vi "Write to DB.vi"(8 "error in (no error)":errorcluster, 11 "Database Entry in":refnum<class "Database Entry.lvclass">) -> (0 "error out":errorcluster, 2 "Stack names":string[](array[string]), 3 "Database Entry out":refnum<class "Database Entry.lvclass">)   [LabVIEW 2021, in "Database Entry.lvclass"]
uses:
  Database Entry.lvclass
  Database Entry.lvclass/Database Entry.ctl
  <vilib>/Utility/file.llb/Read Delimited Spreadsheet (string).vi
  <vilib>/Utility/file.llb/Write Delimited Spreadsheet (string).vi
  Components/Stack/Stack.lvclass
panel:
  out "Final name":string
  out "Data cluster":T1={"module or proto"="proto", " geometry"="full", "resolution"="LD", "baselayer"="BA_123", "toplayer"="SI_789", "bl_pos"="1", "tl_pos"="1", "put_pos"="1", "region"="1", "asstray"="1", "comptray"="1", "put"="1", "date"="2024-04-02", "timestart"="1:12:12.442", "timeend"="1:23:45.244", "operator"="cmuperson", "tape"="some", "glue"="some", "stack name"="some", "Adhesive type"="", "Comments"="", "Temperature"="", "Relative Humidity"=""}
  out "error out py":errorcluster
  out "String Out":string="Upload Success"
  in  "error in (no error) py":errorcluster
  # "Debug instructions\n#### The order of values in db_data_cols must match the order of values in Data cluster in Stack.lvclass: Get stack data.vi \n#### The variable names below correspond to postgres col name. LV does not neet to match the col numes but just the values. \n#### Right-click on the Data cluster on the front panel and click on 'reorder controls' to verify the order is correct in the code. \n#### The physical position of the fields is different from the actual position.\n\nIn Main VIs/python_db/postgres_tools.py, see functions 'assembly_data' and 'assembly_data_as_list'."
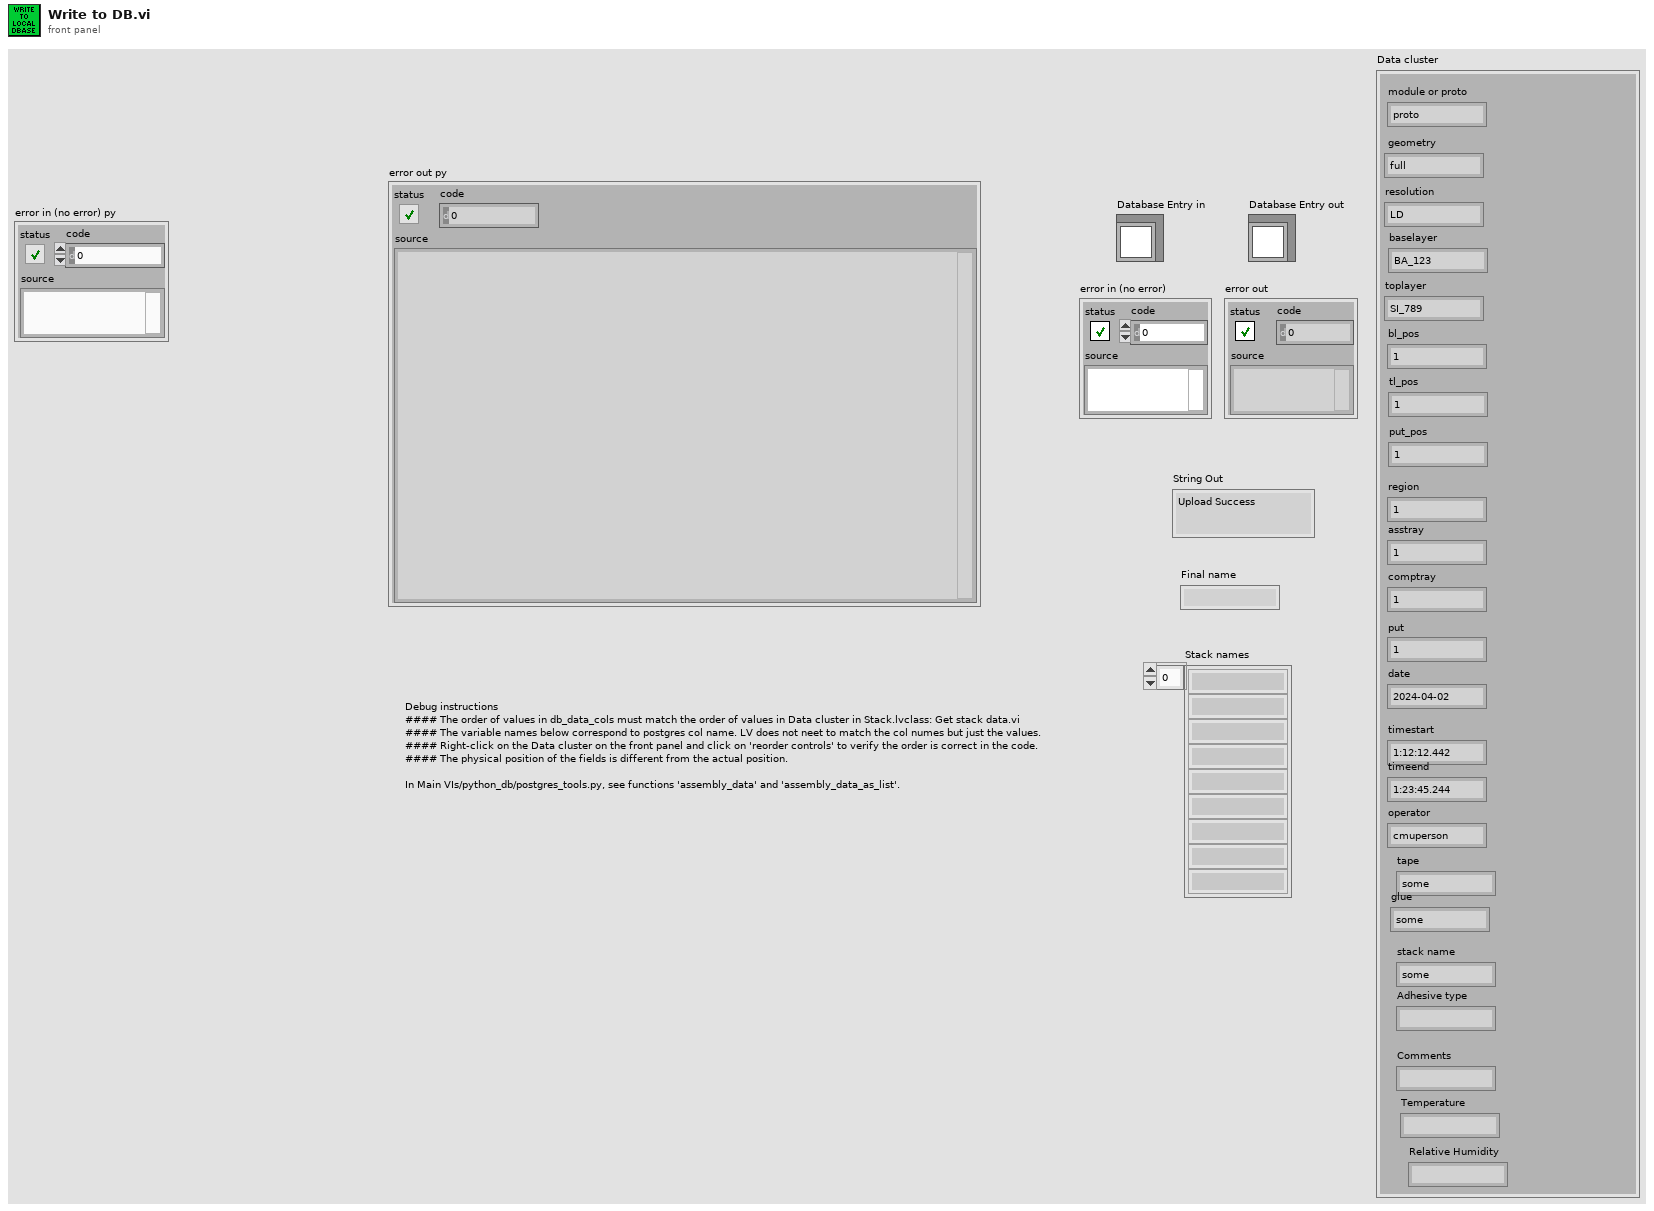
[diagram p1: front panel]
types:
  T1 = cluster{"module or proto":string, " geometry":string, "resolution":string, "baselayer":string, "toplayer":string, "bl_pos":string, "tl_pos":string, "put_pos":string, "region":string, "asstray":string, "comptray":string, "put":string, "date":string, "timestart":string, "timeend":string, "operator":string, "tape":string, "glue":string, "stack name":string, "Adhesive type":string, "Comments":string, "Temperature":string, "Relative Humidity":string}
  T2 = typedef "File Paths.ctl" = cluster{"Glue Pattern Folder":path, "Carrier Tray Folder":path, "Pick Up Tool Fixture Folder":path, "Components Folder":path, "Bellows Tool Offset.txt":path, "Pick Up Tool Offset.txt":path, "Dispense Tip Offset.txt":path, "Log Files":path, "Gantry Assembly Map.txt":path, "Syringe and offset map.txt":path, "Controllers Folder":path, "Local dbase config":path}
  T3 = cluster{"type (proto/module)":string, " geometry":string, "resolution":string, "baselayer":string, "toplayer":string, "bl_pos":string, "tl_pos":string, "put_pos":string, "region":string, "asstray":string, "comptray":string, "put":string, "date":string, "timestart":string, "timeend":string, "operator":string, "tape":string, "glue":string, "stack name":string, "Adhesive type":string, "Comments":string, "Temperature":string, "Relative Humidity":string}
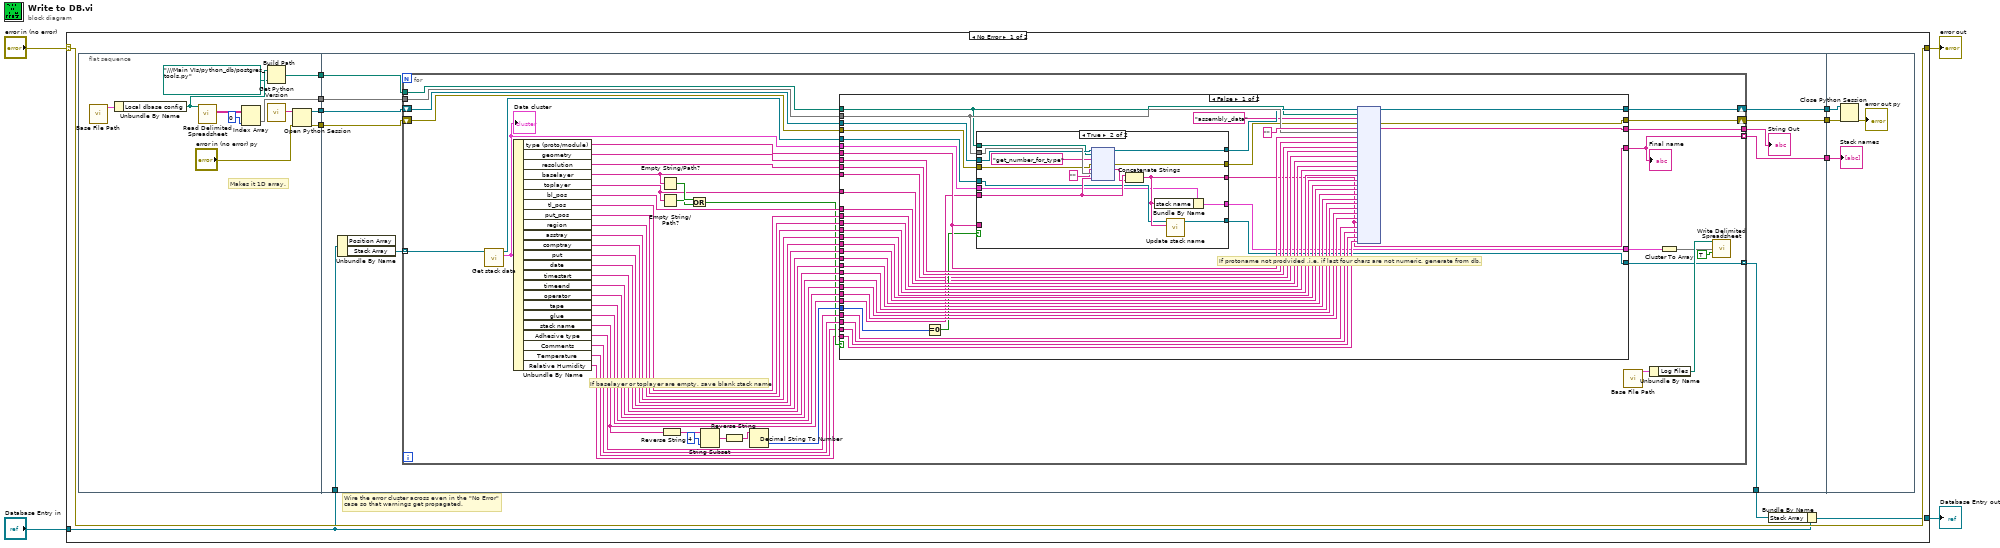
[diagram p0: block diagram]
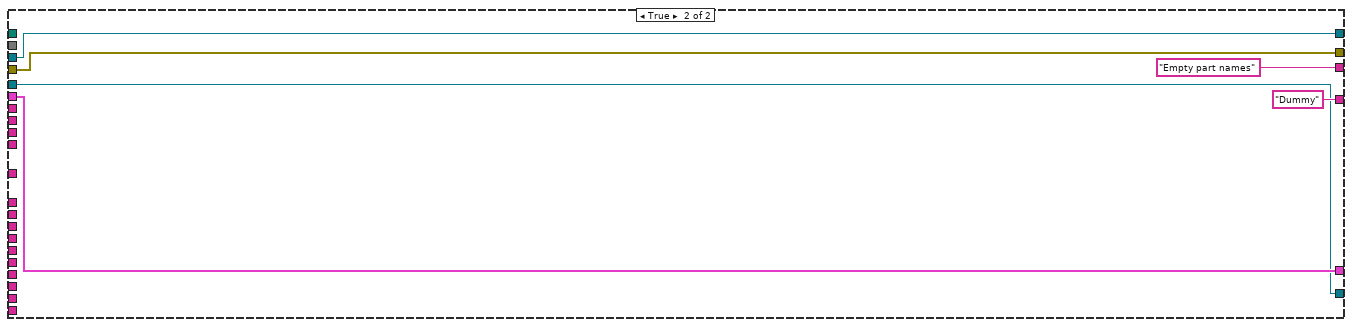
[diagram p3: hidden frame]
diagram:
  n1 = case shown="No Error" "error in (no error)" {
    selector: "error in (no error)" -> [w15 w158]
    tunnel: [w15 w158] -> w3
    tunnel: [w7 w157] -> w1
    tunnel: "Database Entry in" -> [w6 w157]
    frame No Error {
      # "Wire the error cluster across even in the \"No Error\"\ncase so that warnings get propagated."
      n2 = flat-sequence {
        tunnel: [w25] -> w14
        tunnel: [w26] -> w13
        tunnel: [w22] -> w12
        tunnel: [w18] -> w11
        tunnel: [w36] -> w10
        tunnel: [w35] -> w9
        tunnel: w14 -> [w37]
        tunnel: w13 -> [w34]
        tunnel: w12 -> [w33]
        tunnel: w11 -> [w32]
        tunnel: w6 -> [w31]
        tunnel: [w28] -> w8
        tunnel: [w27] -> w5
        tunnel: w10 -> [w155]
        tunnel: w9 -> [w156]
        tunnel: w8 -> [w153]
        frame #0 {
          # "Makes it 1D array."
          n3 = call "Base File Path.vi"() -> ("Paths Out"=w23:T2)  [unwired: 11 in]
          n4 = Unbundle By Name(w23) -> ("Local dbase config"=w21:path)
          n5 = call-poly <vilib>:"Read Delimited Spreadsheet.vi"("file path (dialog if empty)"=w21) -> ("all rows"=w20:string[][])  [unwired: 9 in, 5 out]
          n6 = Index Array(array=w20, index (col)=0 ("disabled index (col)")) -> (element=w18:string[])  [unwired: 1 in]
          n7 = Build Path(base path=w21, name or relative path=path "../../../Main VIs/python_db/postgres_tools.py" ("module path")) -> (appended path=w22:path)
          n8 = call "Get Python Version.vi"() -> ("Python Version"=w16:string)  [unwired: 10 in, 1 out]
          n9 = Open Python Session(python version=w16, 3:"error in (no error) py") -> (session out=w26:refnum<k35>, error out=w25:errorcluster)  [unwired: 1 in]
        }
        frame #1 {
          n10 = Unbundle By Name(w31) -> ("Stack Array"=w29:refnum<class "Stack.lvclass">[])  [unwired: 1 out]
          n11 = for {
            tunnel: w33 -> [w62]
            shift-right: [w85] -> w36
            shift-left: w37 -> [w61]
            shift-right: [w84] -> w35
            shift-left: w34 -> [w63]
            tunnel: [w83] -> w30
            tunnel: w29 -> [w82] mode=indexing
            tunnel: w32 -> [w64]
            tunnel: [w47] -> w28 mode=indexing
            tunnel: [w38] -> w27 mode=indexing
            # "If baselayer or toplayer are empty, save blank stack name"
            n12 = call "Get stack data.vi"("Stack in"=w82) -> ("Data cluster"=w41:T3, "Stack out"=w39:refnum<class "Stack.lvclass">)  [unwired: 8 in, 1 out]
            "Data cluster" <- w41
            n13 = Unbundle By Name(w41) -> ("type (proto/module)"=w65:string, "geometry"=w81:string, "resolution"=w80:string, "baselayer"=w51:string, "toplayer"=w49:string, "bl_pos"=w79:string, "tl_pos"=w78:string, "put_pos"=w77:string, "region"=w60:string, "asstray"=w76:string, "comptray"=w75:string, "put"=w74:string, "date"=w73:string, "timestart"=w72:string, "timeend"=w71:string, "operator"=w70:string, "tape"=w69:string, "glue"=w68:string, "stack name"=w52:string, "Adhesive type"=w59:string, "Comments"=w58:string, "Temperature"=w45:string, "Relative Humidity"=w44:string)
            n14 = Empty String/Path?(string/path=w51) -> (empty?=w50:bool)
            n15 = Empty String/Path?(string/path=w49) -> (empty?=w48:bool)
            n16 = Reverse String(1:w52) -> (0:w57:string)
            n17 = Or(x=w50, y=w48) -> (x .or. y?=w46:bool)
            n18 = String Subset(string=w57, length (rest)=4 ("length (rest)")) -> (substring=w55:string)  [unwired: 1 in]
            n19 = Reverse String(1:w55) -> (0:w54:string)
            n20 = Decimal String To Number(string=w54) -> (number=w53:i32)  [unwired: 2 in, 1 out]
            n21 = case shown="False" w46 {
              tunnel: [w126 w151] -> w85
              tunnel: [w125 w152] -> w84
              tunnel: [w124 "Empty part names"] -> w83
              tunnel: w81 -> [w122 _]
              tunnel: w80 -> [w121 _]
              tunnel: w79 -> [w120 _]
              tunnel: w78 -> [w119 _]
              tunnel: w77 -> [w118 _]
              tunnel: w76 -> [w117 _]
              tunnel: w75 -> [w116 _]
              tunnel: w74 -> [w115 _]
              tunnel: w73 -> [w114 _]
              tunnel: w72 -> [w113 _]
              tunnel: w71 -> [w112 _]
              tunnel: w70 -> [w111 _]
              tunnel: w69 -> [w110 _]
              tunnel: w68 -> [w109 _]
              tunnel: w65 -> [w108 _]
              tunnel: w64 -> [w107 _]
              tunnel: w63 -> [w106 w152]
              tunnel: w62 -> [w104 _]
              tunnel: w61 -> [w103 w151]
              tunnel: w60 -> [w100 _]
              tunnel: w59 -> [w99 _]
              tunnel: w58 -> [w98 _]
              tunnel: w53 -> [w97 _]
              tunnel: w52 -> [w96 _]
              tunnel: w51 -> [w94 _]
              tunnel: w49 -> [w93 _]
              tunnel: [w90 "Dummy" ("stack name")] -> w47
              tunnel: w45 -> [w92 _]
              tunnel: w44 -> [w91 _]
              tunnel: w41 -> [w87 w148]
              tunnel: [w86 w148] -> w40
              tunnel: w39 -> [w88 w147]
              tunnel: [w89 w147] -> w38
              frame False {
                # "If protoname not prodvided ,i.e. if last four chars are not numeric, generate from db."
                n22 = Equal To 0?(x=w97) -> (x = 0?=w95:bool)
                n23 = case shown="True" w95 {
                  tunnel: w108 -> [_ _]
                  tunnel: w96 -> [w129 w146]
                  tunnel: w107 -> [_ w145]
                  tunnel: w106 -> [w131 w144]
                  tunnel: [w131 w143] -> w105
                  tunnel: w104 -> [_ w142]
                  tunnel: w103 -> [w130 w141]
                  tunnel: [w130 w140] -> w102
                  tunnel: [w129 w139] -> w90
                  tunnel: [w128 w135] -> w89
                  tunnel: w88 -> [w128 w134]
                  tunnel: w87 -> [w127 w133]
                  tunnel: [w127 w132] -> w86
                  frame False {
                  }
                  frame True {
                    n24 = node(w144, w142, "get_number_for_type" ("function name"), w141, "" ("function name"), w145, w146) -> (w143:refnum<k35>, w140:errorcluster, w136:string)  [unwired: 2 in, 2 out]
                    n25 = Concatenate Strings(w146, w136) -> (w139:string)
                    n26 = Bundle By Name(cluster=w133, "stack name"=w139) -> (w132:T3)
                    n27 = call "Update stack name.vi"("Stack ID updated"=w139, "Stack in"=w134) -> ("Stack out"=w135:refnum<class "Stack.lvclass">)  [unwired: 8 in, 1 out]
                  }
                }
                n28 = node(w105, w104, "assembly_data" ("function name"), w102, "", w107, w108, w122, w121, w94, w93, w120, w119, w118, w100, w117, w116, w115, w114, w113, w112, w111, w110, w109, w90, w99, w98, w92, w91) -> (w125:refnum<k35>, w126:errorcluster, w124:string)  [unwired: 24 in, 2 out]
              }
              frame True {
              }
            }
            "Final name" <- w47
            n29 = call "Base File Path.vi"() -> ("Paths Out"=w67:T2)  [unwired: 11 in]
            n30 = Unbundle By Name(w67) -> ("Log Files"=w66:path)
            n31 = Cluster To Array(cluster=w40) -> (array=w42:string[])
            n32 = call-poly <vilib>:"Write Delimited Spreadsheet.vi"("file path (dialog if empty)"=w66, "1D data"=w42, "append to file? (new file:F)"=TRUE) -> ()  [unwired: 11 in, 2 out]
          }
          "String Out" <- w30
        }
        frame #2 {
          n33 = Close Python Session(session in=w156, error in=w155) -> (11:→"error out py":errorcluster)
          "Stack names" <- w153
        }
      }
      n34 = Bundle By Name(cluster=w6, "Stack Array"=w5) -> (w7:refnum<class "Database Entry.lvclass">)
    }
    frame Error {
    }
  }
  "error out" <- w3
  "Database Entry out" <- w1
